vi "SV TDMS Write XY (1 Ch).vi"(0 "tdms file":refnum<k34>, 2 "write mode":u16(ring) items=["Append", "New group", "Overwrite"], 5 "group name in":string="XY", 7 "channel name in":string="Channel0", 9 "XY":cluster{"X":dbl[], "Y":dbl[]}, 11 "error in":errorcluster, 12 "unit info":T5, 13 "function info":T4={"function type"=0, "function subtype"=2, "X-dimension"=0} {"X-dimension" items=["Time (s)"=0, "Frequency-CB (Hz)"=1, "Frequency-CPB (Hz)"=1248, "Frequency-Arbitrary (Hz)"=2357, "Quefrency (s)"=2, "Revolutions (rev)"=3, "Order"=4, "Speed (RPM)"=11, "Speed (rad/s)"=21, "Index"=65535]; "function subtype" items=["Unscaled binary"=0, "Scaled voltage"=1, "Scaled engineering units"=2, "-"=10, "Value"=19, "DC"=11, "AC"=12, "RMS^2"=13, "RMS"=14, "Peak"=15, "Peak to peak"=16, "-"=20, "1/1 octave"=21, "1/3 octave"=22, "1/6 octave"=23, "1/12 octave"=24, "1/24 octave"=25, "-"=30, "Density"=31, "Magnitude"=32, "Phase"=33, "Real"=34, "Imaginary"=35, "Complex"=345, "Coherence"=36, "-"=90, "Unknown"=99]; "function type" items=["Signal"=0, "Speed"=3, "Ratio"=6, "Count"=7, "-"=9, "Level"=10, "-"=19, "Octave Spectrum"=20, "-"=29, "FFT Auto Spectrum"=30, "FFT Cross Spectrum"=40, "Frequency Response"=50, "-"=59, "Event"=90]}) -> (4 "tdms file out":refnum<k34>, 6 "group name out":string, 8 "channel name out":string, 15 "error out":errorcluster)   [LabVIEW 2017]
uses:
  <vilib>/addons/_NISVFA/_Shared subVIs/Controls/NI Function Type.ctl
  <vilib>/addons/_NISVFA/_Shared subVIs/Controls/NI Function SubType.ctl
  <vilib>/addons/_NISVFA/_Shared subVIs/Controls/svc_X-Axis Units.ctl
  <vilib>/addons/_NISVFA/_Shared subVIs/Controls/LV Datatypes.ctl
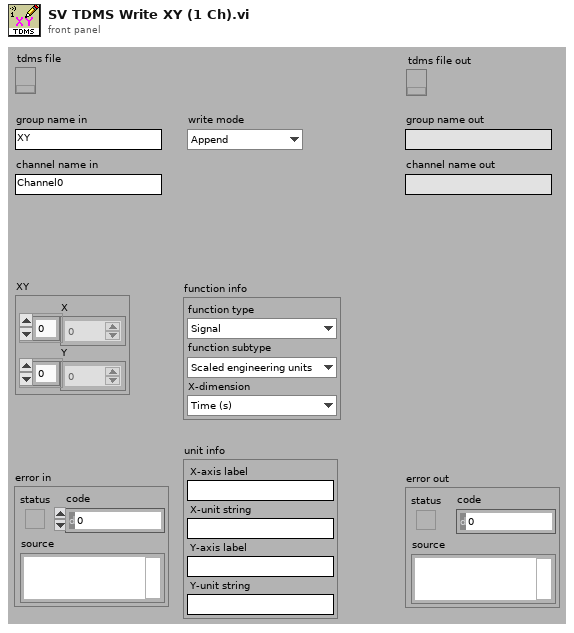
[diagram p1: front panel]
types:
  T1 = typedef "NI Function Type.ctl" = u16
  T2 = typedef "NI Function SubType.ctl" = u16
  T3 = typedef "svc_X-Axis Units.ctl" = u16
  T4 = cluster{"function type":T1, "function subtype":T2, "X-dimension":T3}
  T5 = cluster{"X-axis label":string, "X-unit string":string, "Y-axis label":string, "Y-unit string":string}
  T6 = typedef "LV Datatypes.ctl" = i32
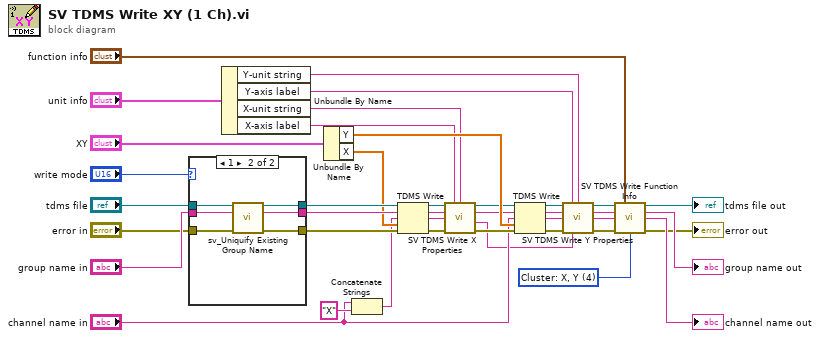
[diagram p0: block diagram]
diagram:
  w12 = T6 4 items=["String: abc"=-2, "Boolean: True or False"=-1, "Scalar: y"=0, "Array: Y"=1, "Waveform: t0, dt, Y, variant"=2, "Cluster: x0, dx, Y"=3, "Cluster: X, Y"=4, "Waterfall"=5, "Colormap"=6] ("LabVIEW datatype")
  n1 = case shown="1" "write mode" {
    tunnel: [w43 w46] -> w40
    tunnel: [w41 w44] -> w39
    tunnel: "group name in" -> [w41 w45]
    tunnel: [w42 w47] -> w36
    tunnel: "error in" -> [w42 w48]
    tunnel: "tdms file" -> [w43 w49]
    frame 0, Default {
    }
    frame 1 {
      n2 = call <vilib>:"sv_Uniquify Existing Group Name.vi"("tdms file ref"=w49, "group name"=w45, "error in"=w48) -> ("tdms file out"=w46:refnum<k34>, "unique group"=w44:string, "error out"=w47:errorcluster)  [unwired: 10 in]
    }
  }
  n3 = Unbundle By Name("unit info") -> ("Y-unit string"=w10:string, "Y-axis label"=w11:string, "X-unit string"=w27:string, "X-axis label"=w22:string)
  n4 = Unbundle By Name("XY") -> ("Y"=w33:dbl[], "X"=w37:dbl[])
  n5 = Concatenate Strings("channel name in", "X" ("string")) -> (w18:string)
  n6 = TDMS Write(0:w40, 5:w39, 7:w18, 9:w37, 11:w36) -> (4:w23:refnum<k34>, 6:w24:string, 8:w25:string, 15:w26:errorcluster)  [unwired: 1 in]
  n7 = call <vilib>:"SV TDMS Write X Properties.vi"("tdms file in"=w23, "X-axis label"=w22, "X-unit string"=w27, "group name"=w24, "channel name"=w25, "error in"=w26) -> ("tdms file out"=w31:refnum<k34>, "group name"=w29:string, "channel name"=w1:string, "error out"=w30:errorcluster)  [unwired: 6 in]
  n8 = TDMS Write(0:w31, 5:w29, 7:"channel name in", 9:w33, 11:w30) -> (4:w9:refnum<k34>, 6:w8:string, 8:w7:string, 15:w6:errorcluster)  [unwired: 1 in]
  n9 = call <vilib>:"SV TDMS Write Y Properties.vi"("tdms file"=w9, "y-axis label"=w11, "y-unit string"=w10, "group name"=w8, "channel name"=w7, "error in (no error)"=w6, "xchannel name"=w1) -> ("tdms file out"=w2:refnum<k34>, "group name"=w3:string, "channel name"=w4:string, "error out"=w5:errorcluster)  [unwired: 5 in]
  n10 = call <vilib>:"SV TDMS Write Function Info.vi"("tdms file in"=w2, "function info"="function info", "LabVIEW datatype"=w12, "group name"=w3, "channel name"=w4, "error in (no error)"=w5) -> ("tdms file out"=→"tdms file out":refnum<k34>, "group name out"=→"group name out":string, "channel name out"=→"channel name out":string, "error out"=→"error out":errorcluster)  [unwired: 6 in]
